vi "Measuring Complete - AndreTec-5-2.vi"() -> ()   [LabVIEW 2014]
doc: "André Romero - 2016\nandretec@ifsc.usp.br\nIFSC - USP"
uses:
  <vilib>/Analysis/Matrix/Datatypes/RealMatrix.ctl
  <vilib>/Analysis/Matrix/NI_Matrix.lvlib
  <vilib>/Instr/_visa.llb/VISA Configure Serial Port (Instr).vi
  <vilib>/Utility/file.llb/Write To Spreadsheet File (DBL).vi
  C:/UserLabs/Andre/Nova-Autolab/Labview/Autolab SDK 1.11/EcoChemie.Autolab.Sdk.dll
  EcoChemie.Autolab.Sdk.dll
panel:
  out "Procedure array":path[](array[path])=[path "C:/Users/user/Documents/My Procedures 1.11/Procedures/bla.nox", path "C:/Users/user/Documents/My Procedures 1.11/Procedures/bla2.nox", path "", path "", path "", path "", path "", path ""]
  in  "Tab Control":enum32{"Settings", "Measuring..."}(tab)
  in  "Load Procedure #8":path
  in  "Load Procedure #7":path
  in  "Load Procedure #6":path
  in  "Load Procedure #5":path
  in  "Load Procedure #4":path
  in  "Load Procedure #3":path
  in  "Load Procedure #2":path=path "C:/Users/user/Documents/My Procedures 1.11/Procedures/bla2.nox"
  in  "Load Procedure #1":path=path "C:/Users/user/Documents/My Procedures 1.11/Procedures/bla.nox"
  in  "Start Measurement":bool
  in  "X axis Sensor 1":string(combo)="WE(1).Potential"
  in  "Y axis Sersor 1":string(combo)="WE(1).Current"
  in  "X axis Sensor 2":string(combo)="WE(1).Potential"
  in  "Y axis Sersor 2":string(combo)="WE(1).Current"
  in  "X axis Sensor 3":string(combo)="WE(1).Potential"
  in  "Y axis Sersor 3":string(combo)="WE(1).Current"
  in  "X axis Sensor 4":string(combo)="WE(1).Potential"
  in  "Y axis Sersor 4":string(combo)="WE(1).Current"
  in  "X axis Sensor 5":string(combo)="WE(1).Potential"
  in  "Y axis Sersor 5":string(combo)="WE(1).Current"
  in  "X axis Sensor 6":string(combo)="WE(1).Potential"
  in  "Y axis Sersor 6":string(combo)="WE(1).Current"
  in  "X axis Sensor 7":string(combo)="WE(1).Potential"
  in  "Y axis Sersor 7":string(combo)="WE(1).Current"
  in  "X axis Sensor 8":string(combo)="WE(1).Potential"
  in  "Y axis Sersor 8":string(combo)="WE(1).Current"
  out "Measured data":cluster{"Y":dbl[], "Y":dbl[]}[](graph)=[{"Y"=[7.324218750000278e-05, 7.324218750000278e-05, 7.324218750000278e-05, 7.324218750000278e-05, 7.324218750000278e-05, 7.324218750000278e-05, 7.324218750000278e-05, 7.324218750000278e-05, 7.324218750000278e-05, 7.324218750000278e-05, 7.324218750000278e-05, 7.324218750000278e-05, 7.324218750000278e-05, 7.324218750000278e-05, 7.324218750000278e-05, 7.324218750000278e-05, 7.324218750000278e-05, 7.324218750000278e-05, 7.324218750000278e-05, 7.324218750000278e-05, 7.324218750000278e-05, 7.324218750000278e-05, 7.324218750000278e-05, 7.324218750000278e-05, 7.324218750000278e-05, 7.324218750000278e-05, 7.324218750000278e-05, 7.324218750000278e-05, 7.324218750000278e-05, 7.324218750000278e-05, 7.324218750000278e-05, 7.324218750000278e-05, 3.967285156250555e-05, 0.007351684570312503, 0.0195159912109375, 0.026904296874999997, 0.039157104492187504, 0.048931884765625, 0.06103515625, 0.068450927734375, 0.078125, 0.095245361328125, 0.10504150390625, 0.114776611328125, 0.1246337890625, 0.1343994140625, 0.144134521484375, 0.156402587890625, 0.163787841796875, 0.173431396484375, 0.185821533203125, 0.193084716796875, 0.205322265625, 0.215057373046875, 0.224945068359375, 0.234649658203125, 0.244384765625, 0.254180908203125, 0.266448974609375, 0.27386474609375, 0.285980224609375, 0.293365478515625, 0.30560302734375, 0.315277099609375, 0.32525634765625, 0.33502197265625, 0.347259521484375, 0.354461669921875, 0.364288330078125, 0.3765869140625, 0.38623046875, 0.396148681640625, 0.40594482421875, 0.415618896484375, 0.42791748046875, 0.435302734375, 0.447540283203125, 0.45477294921875, 0.467041015625, 0.474395751953125, 0.4864501953125, 0.4864501953125, 0.4864501953125, 0.4864501953125, 0.4864501953125, 0.4864501953125, 0.4864501953125, 0.4864501953125, 0.4864501953125, 0.4864501953125, 0.4864501953125, 0.4864501953125, 0.4864501953125, 0.4864501953125, 0.4864501953125, 0.4864501953125, 0.4864501953125, 0.4864501953125, 0.4864501953125, 0.4864501953125, 0.4864501953125, 0.4864501953125, 0.4864501953125, 0.4864501953125, 0.4864501953125, 0.4864501953125, 0.4864501953125, 0.4864501953125, 0.4864501953125, 0.4864501953125, 0.4864501953125, 0.4864501953125, 0.4864501953125, 0.4864501953125, 0.4864501953125, 0.4864501953125, 0.4864501953125, 0.4864501953125, 0.4864501953125, 0.4864501953125, 0.4864501953125, 0.4864501953125, 0.4864501953125, 0.4864501953125, 0.4864501953125, 0.4864501953125], "Y"=[-1.5228271484375027e-09, -1.5228271484375027e-09, -1.5228271484375027e-09, -1.5228271484375027e-09, -1.5228271484375027e-09, -1.5228271484375027e-09, -1.5228271484375027e-09, -1.5228271484375027e-09, -1.5228271484375027e-09, -1.5228271484375027e-09, -1.5228271484375027e-09, -1.5228271484375027e-09, -1.5228271484375027e-09, -1.5228271484375027e-09, -1.5228271484375027e-09, -1.5228271484375027e-09, -1.5228271484375027e-09, -1.5228271484375027e-09, -1.5228271484375027e-09, -1.5228271484375027e-09, -1.5228271484375027e-09, -1.5228271484375027e-09, -1.5228271484375027e-09, -1.5228271484375027e-09, -1.5228271484375027e-09, -1.5228271484375027e-09, -1.5228271484375027e-09, -1.5228271484375027e-09, -1.5228271484375027e-09, -1.5228271484375027e-09, -1.5228271484375027e-09, -1.5228271484375027e-09, 1.2298583984375e-09, 8.026123046875e-09, 2.056884765625e-08, 2.8045654296875e-08, 4.3182373046875e-08, 5.0750732421875e-08, 6.0791015625e-08, 7.302856445312499e-08, 8.0780029296875e-08, 9.7625732421875e-08, 1.02691650390625e-07, 1.1566162109375e-07, 1.23779296875e-07, 1.3873291015625e-07, 1.4031982421875e-07, 1.5744018554687499e-07, 1.6473388671875e-07, 1.7724609375e-07, 1.8524169921875e-07, 1.97265625e-07, 2.03948974609375e-07, 2.15118408203125e-07, 2.2833251953125e-07, 2.3315429687499998e-07, 2.47528076171875e-07, 2.5543212890624997e-07, 2.6641845703125e-07, 2.72979736328125e-07, 2.86376953125e-07, 2.97393798828125e-07, 3.0657958984375e-07, 3.16162109375e-07, 3.27911376953125e-07, 3.33251953125e-07, 3.4716796874999997e-07, 3.55987548828125e-07, 3.6611938476562497e-07, 3.74664306640625e-07, 3.900146484375e-07, 3.9682006835937497e-07, 4.1180419921874997e-07, 4.16595458984375e-07, 4.2974853515624997e-07, 4.3438720703125e-07, 4.505615234375e-07, 4.55657958984375e-07, 4.6716308593749996e-07, 4.7686767578125e-07, 4.91546630859375e-07, 4.91546630859375e-07, 4.91546630859375e-07, 4.91546630859375e-07, 4.91546630859375e-07, 4.91546630859375e-07, 4.91546630859375e-07, 4.91546630859375e-07, 4.91546630859375e-07, 4.91546630859375e-07, 4.91546630859375e-07, 4.91546630859375e-07, 4.91546630859375e-07, 4.91546630859375e-07, 4.91546630859375e-07, 4.91546630859375e-07, 4.91546630859375e-07, 4.91546630859375e-07, 4.91546630859375e-07, 4.91546630859375e-07, 4.91546630859375e-07, 4.91546630859375e-07, 4.91546630859375e-07, 4.91546630859375e-07, 4.91546630859375e-07, 4.91546630859375e-07, 4.91546630859375e-07, 4.91546630859375e-07, 4.91546630859375e-07, 4.91546630859375e-07, 4.91546630859375e-07, 4.91546630859375e-07, 4.91546630859375e-07, 4.91546630859375e-07, 4.91546630859375e-07, 4.91546630859375e-07, 4.91546630859375e-07, 4.91546630859375e-07, 4.91546630859375e-07, 4.91546630859375e-07, 4.91546630859375e-07, 4.91546630859375e-07, 4.91546630859375e-07, 4.91546630859375e-07, 4.91546630859375e-07, 4.91546630859375e-07]}]
  out "Autolab Connected":bool
  out "Blacklisted Commands detected":bool
  out "Y axis value":dbl=4.91546630859375e-07
  out "X axis value":dbl=0.4864501953125
  in  "X axis Signal":string(combo)="WE(1).Potential"
  in  "Y axis Signal":string(combo)="WE(1).Current"
  out "Points":i32=30
  out "Sensor":i32=2
  out "Measurement active":bool
  in  "Abort":bool
  in  "String":string="Wait !!!! Instrument is initializing ...."
  out "Measurement":cluster{dbl[], dbl[]}(graph)={[0.4864501953125, 0.4864501953125, 0.4864501953125, 0.4864501953125, 0.4864501953125, 0.4864501953125, 0.4864501953125, 0.4864501953125, 0.4864501953125, 0.4864501953125, 0.4864501953125, 0.4864501953125, 0.4864501953125, 0.4864501953125, 0.4864501953125, 0.4864501953125, 0.4864501953125, 0.4864501953125, 0.4864501953125, 0.4864501953125, 0.4864501953125, 0.4864501953125, 0.4864501953125, 0.4864501953125, 0.4864501953125, 0.4864501953125, 0.4864501953125, 0.4864501953125, 0.4864501953125, 0.4864501953125, 0.4864501953125], [4.91546630859375e-07, 4.91546630859375e-07, 4.91546630859375e-07, 4.91546630859375e-07, 4.91546630859375e-07, 4.91546630859375e-07, 4.91546630859375e-07, 4.91546630859375e-07, 4.91546630859375e-07, 4.91546630859375e-07, 4.91546630859375e-07, 4.91546630859375e-07, 4.91546630859375e-07, 4.91546630859375e-07, 4.91546630859375e-07, 4.91546630859375e-07, 4.91546630859375e-07, 4.91546630859375e-07, 4.91546630859375e-07, 4.91546630859375e-07, 4.91546630859375e-07, 4.91546630859375e-07, 4.91546630859375e-07, 4.91546630859375e-07, 4.91546630859375e-07, 4.91546630859375e-07, 4.91546630859375e-07, 4.91546630859375e-07, 4.91546630859375e-07, 4.91546630859375e-07, 4.91546630859375e-07]}
  out "error out":errorcluster
  out "VISA resource name out":refnum<visa-resource-name>="ASRL3::INSTR"
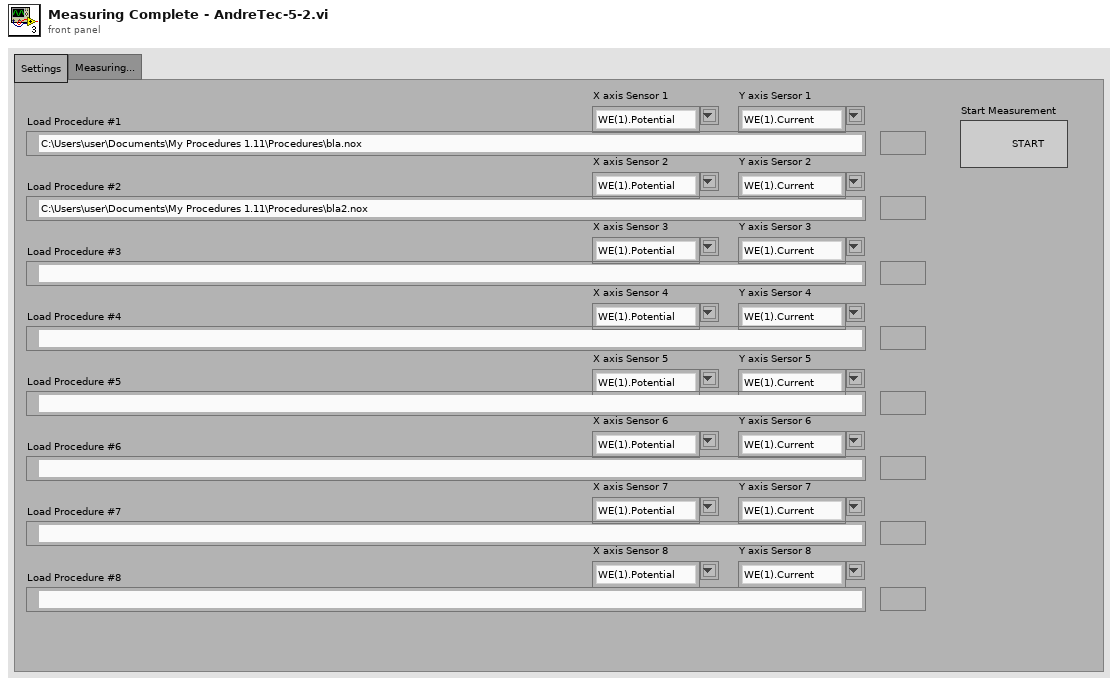
[diagram p1: front panel]
types:
  T1 = typedef "NI_Matrix.lvlib/RealMatrix.ctl" = dbl[][]
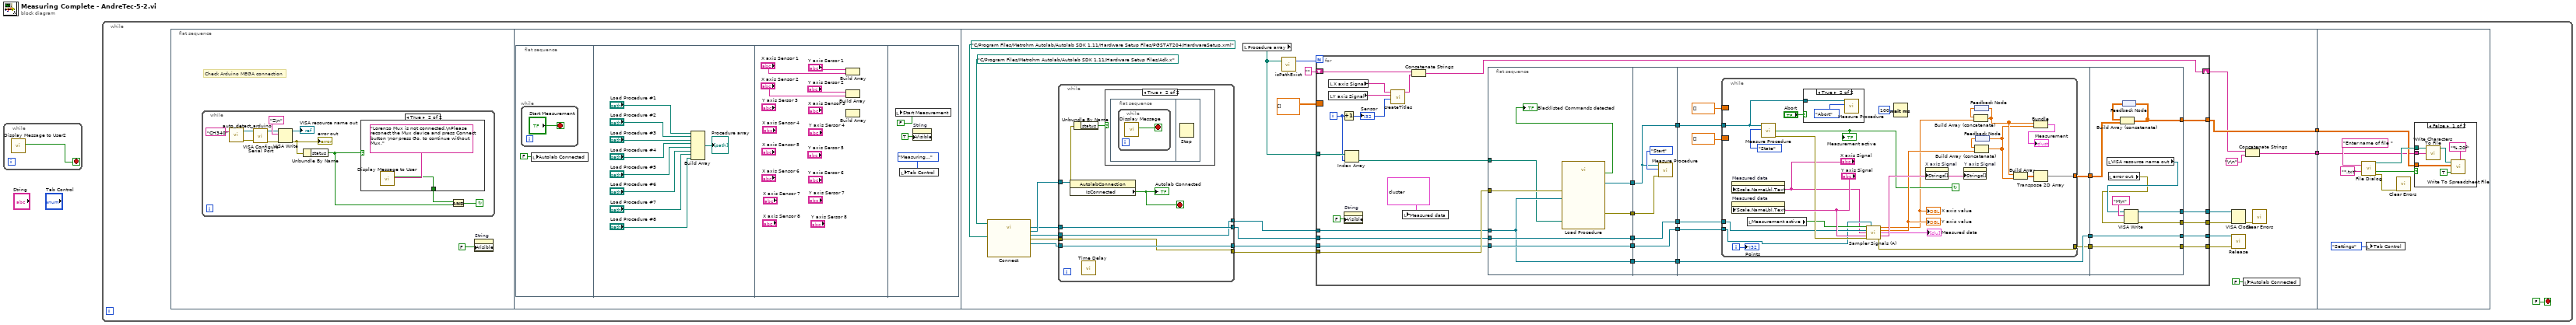
[diagram p0: block diagram]
diagram:
  n1 = while {
    stop <- w1 stop-if-true
    n2 = call "Display Message to User2"() -> ("OK"=w1:bool)  [unwired: 10 in, 1 out]
  }
  n3 = while {
    stop <- FALSE stop-if-true
    n4 = flat-sequence {
      tunnel: [w42] -> w3
      tunnel: [w40] -> w2
      tunnel: w3 -> [w163]
      tunnel: w2 -> [w162]
      frame #0 {
        # "Check Arduino MEGA connection"
        n5 = while {
          stop <- w8 continue-if-true
          n6 = call "auto_detect_arduino.vi"("instr name"="CH340") -> ("VISA resource name"=w16:refnum<visa-resource-name>, "error out"=w9:errorcluster)  [unwired: 1 in, 1 out]
          n7 = call-poly "VISA Configure Serial Port"("VISA resource name"=w16, "error in (no error)"=w9) -> ("VISA resource name out"=w13:refnum<visa-resource-name>, "error out"=w12:errorcluster)  [unwired: 7 in, 5 out]
          n8 = VISA Write(VISA resource name=w13, write buffer="Z\n" ("Command"), error in (no error)=w12) -> (VISA resource name out=→"VISA resource name out":refnum<visa-resource-name>, error out=w10:errorcluster)  [unwired: 1 out]
          "error out" <- w10
          n9 = Unbundle By Name(w10) -> ("status"=w7:bool)
          n10 = case shown="True" w7 {
            tunnel: [_ w17] -> w6
            frame False {
            }
            frame True {
              n11 = call "Display Message to User"("Message"="Lorenzo Mux is not connected.\nPlease reconect the Mux device and press Connect button \nor press Go, to continue without Mux.") -> ("Connect"=w17:bool)  [unwired: 9 in, 1 out]
            }
          }
          n12 = And(x=w6, y=w7) -> (x .and. y?=w8:bool)
        }
        n13 = property on="String" class="Str"("Visible"=FALSE) -> ()  [unwired: 2 in, 2 out]
      }
      frame #1 {
        n14 = flat-sequence {
          frame #0 {
            n15 = while {
              stop <- "Start Measurement" stop-if-true
            }
            n16 = local write "Autolab Connected"(FALSE ("Autolab Connected")) -> ()
          }
          frame #1 {
            n17 = Build Array("Load Procedure #1", "Load Procedure #2", "Load Procedure #3", "Load Procedure #4", "Load Procedure #5", "Load Procedure #6", "Load Procedure #7", "Load Procedure #8") -> (→"Procedure array":path[])
          }
          frame #2 {
            n18 = Build Array("Y axis Sersor 2", "X axis Sensor 2") -> ()  [unwired: 1 out]
            n19 = Build Array("Y axis Sersor 1", "X axis Sensor 1") -> ()  [unwired: 1 out]
            n20 = Build Array() -> ()  [unwired: 2 in, 1 out]
          }
          frame #3 {
            n21 = local write "Start Measurement"(FALSE ("Start Measurement")) -> ()
            n22 = local write "Tab Control"(enum32{"Settings", "Measuring..."}."Measuring..." ("Tab Control")) -> ()
            n23 = property on="String" class="Str"("Visible"=TRUE) -> ()  [unwired: 2 in, 2 out]
          }
        }
      }
      frame #2 {
        n24 = call "Connect.vi"("Embedded Exe File"=path "C:/Program Files/Metrohm Autolab/Autolab SDK 1.11/Hardware Setup Files/Adk.x", "Hardware Setup File"=path "C:/Program Files/Metrohm Autolab/Autolab SDK 1.11/Hardware Setup Files/PGSTAT204/HardwareSetup.xml") -> ("Sampler"=w58:refnum<k24>, "AutolabConnection"=w59:refnum<k24>, "instrument"=w56:refnum<k24>, "Ei"=w51:refnum<k24>, "error out"=w53:errorcluster)  [unwired: 1 in, 8 out]
        n25 = while {
          tunnel: w59 -> [w158]
          tunnel: w58 -> [w155]
          tunnel: [w155] -> w57
          tunnel: w56 -> [w154]
          tunnel: [w154] -> w55
          tunnel: w51 -> [w153]
          tunnel: [w153] -> w54
          tunnel: w53 -> [w152]
          tunnel: [w152] -> w52
          stop <- w159 stop-if-true
          n26 = property class="AutolabConnection"(reference=w158) -> (error out=w156:errorcluster, "IsConnected"=w159:bool)  [unwired: 1 in, 1 out]
          "Autolab Connected" <- w159
          n27 = Unbundle By Name(w156) -> ("status"=w157:bool)
          n28 = call "Time Delay"() -> ()  [unwired: 2 in, 10 out]
          n29 = case shown="True" w157 {
            frame False {
            }
            frame True {
              n30 = flat-sequence {
                frame #0 {
                  n31 = while {
                    stop <- w160 stop-if-true
                    n32 = call "Display Message"() -> ("OK"=w160:bool)  [unwired: 10 in, 1 out]
                  }
                }
                frame #1 {
                  n33 = Stop() -> ()  [unwired: 1 in]
                }
              }
            }
          }
        }
        n34 = local read "Procedure array"() -> (w37:path[])
        n35 = call "isPathExist.vi"("Array"=w37) -> ("Numeric"=w38:i16)  [unwired: 2 in]
        n36 = for {
          N: w38 -> [_]
          tunnel: [w82] -> w50
          tunnel: [w81] -> w49
          tunnel: [w80] -> w47
          tunnel: [w79] -> w46
          tunnel: w52 -> [w78]
          tunnel: w55 -> [w77]
          tunnel: w57 -> [w76]
          tunnel: w54 -> [w75]
          tunnel: [w73] -> w42
          border: T1 [] ("Real Matrix") -> [_]
          shift-right: [w70] -> w41
          shift-left: "" -> [w71]
          tunnel: w37 -> [w65]
          i -> [w64]
          n37 = local read "Y axis Signal"() -> (w68:string)
          n38 = local read "X axis Signal"() -> (w69:string)
          n39 = Increment(x=w64) -> (x+1=w67:i32)
          "Sensor" <- w67
          n40 = property on="String" class="Str"("Visible"=FALSE) -> ()  [unwired: 2 in, 2 out]
          n41 = Index Array(array=w65, index=w64) -> (element=w63:path)
          n42 = call "createTitles.vi"("Numeric"=w67, "Y axis Signal"=w68, "X axis Signal"=w69) -> ("String"=w66:string)  [unwired: 8 in]
          n43 = local write "Measured data"(cluster{"Y":dbl[], "Y":dbl[]}[] [{"Y"=array[2393 elements], "Y"=array[2393 elements]}] ("Measured data")) -> ()
          n44 = Concatenate Strings(w71, w66) -> (w70:string)
          n45 = flat-sequence {
            tunnel: [w100] -> w93
            tunnel: [w99] -> w92
            tunnel: [w97] -> w91
            tunnel: [w96] -> w90
            tunnel: [w95] -> w89
            tunnel: w77 -> [w95]
            tunnel: w78 -> [w98]
            tunnel: w76 -> [w97]
            tunnel: w75 -> [w96]
            tunnel: w63 -> [w94]
            tunnel: w93 -> [w105]
            tunnel: w92 -> [w106]
            tunnel: [w105] -> w88
            tunnel: w91 -> [w104]
            tunnel: w90 -> [w103]
            tunnel: [w104] -> w87
            tunnel: [w103] -> w86
            tunnel: [w102] -> w85
            tunnel: w89 -> [w102]
            tunnel: w88 -> [w115]
            tunnel: w87 -> [w114]
            tunnel: w86 -> [w113]
            tunnel: w85 -> [w112]
            tunnel: [w112] -> w84
            tunnel: [w108] -> w83
            tunnel: [w111] -> w74
            tunnel: w84 -> [w151]
            tunnel: w83 -> [w150]
            tunnel: [w151] -> w82
            tunnel: [w150] -> w81
            tunnel: [w146] -> w80
            tunnel: [w145] -> w79
            tunnel: w74 -> [w144]
            tunnel: [w142] -> w73
            frame #0 {
              n46 = call "Load Procedure.vi"("error in (no error)"=w98, "Procedure"=w94, "Instrument"=w95) -> ("error out"=w99:errorcluster, "Contains"=→"Blacklisted Commands detected":bool, "LoadProcedure"=w100:refnum<k24>)  [unwired: 6 out]
            }
            frame #1 {
              n47 = call "Measure Procedure.vi"("error in"=w106, "Request for procedure"=enum16{"State", "Save", "Abort", "Start"}."Start", "LoadProcedure"=w105) -> ()  [unwired: 1 in, 8 out]
            }
            frame #2 {
              n48 = while {
                tunnel: w115 -> [w132]
                tunnel: w114 -> [w133]
                tunnel: w113 -> [w117]
                tunnel: [w120] -> w111
                border: dbl[] [] -> [_]
                border: dbl[] [] -> [_]
                tunnel: [w119] -> w108
                i -> [w129]
                stop <- w124 continue-if-true
                n49 = property on="Measured data" class="XYGraph (strict)"("XScale.NameLbl.Text"="X axis Signal") -> ()  [unwired: 2 in, 2 out]
                n50 = property on="Measured data" class="XYGraph (strict)"("YScale.NameLbl.Text"="Y axis Signal") -> ()  [unwired: 2 in, 2 out]
                n51 = local read "Measurement active"() -> (w135:bool)
                n52 = call "Measure Procedure.vi"("Request for procedure"=enum16{"State", "Save", "Abort", "Start"}."State", "LoadProcedure"=w132) -> ("error out"=w136:errorcluster, "IsMeasuring"=w124:bool)  [unwired: 2 in, 6 out]
                "Measurement active" <- w124
                n53 = case shown="True" "Abort" {
                  tunnel: w132 -> [_ w140]
                  frame False {
                  }
                  frame True {
                    n54 = call "Measure Procedure.vi"("Request for procedure"=enum16{"State", "Save", "Abort", "Start"}."Abort", "LoadProcedure"=w140) -> ()  [unwired: 2 in, 8 out]
                  }
                }
                n55 = call "Sampler Signals (A).vi"("IsMeasuring"=w135, "EI"=w117, "Sampler"=w133, "Signal X"="X axis Signal", "Signal Y"="Y axis Signal", "error in"=w136) -> ("X"=w118:dbl, "Y"=w126:dbl, "XY Graph"=→"Measured data":cluster{"Y":dbl[], "Y":dbl[]}[], "GetSignals"=w138:string[], "error out"=w119:errorcluster)  [unwired: 4 in, 1 out]
                "Y axis value" <- w126
                "X axis value" <- w118
                n56 = Wait (ms)(milliseconds to wait=u32 100) -> ()  [unwired: 1 out]
                n57 = property on="X axis Signal" class="CmbBox"("Strings[]"=w138) -> ()  [unwired: 2 in, 2 out]
                n58 = property on="Y axis Signal" class="CmbBox"("Strings[]"=w138) -> ()  [unwired: 2 in, 2 out]
                n59 = feedback #1() -> (w128:dbl[])
                n60 = Build Array (concatenate)(w128, w118) -> (w122:dbl[])
                n61 = feedback-in #1(w122) -> ()
                n62 = feedback #2() -> (w127:dbl[])
                n63 = Build Array (concatenate)(w127, w126) -> (w121:dbl[])
                n64 = feedback-in #2(w121) -> ()
                n65 = Build Array(w122, w121) -> (w123:dbl[][])
                n66 = Bundle(w122, w121) -> (→"Measurement":cluster{dbl[], dbl[]})  [unwired: 1 in]
                n67 = Transpose 2D Array(2D array=w123) -> (transposed array=w120:dbl[][])
                "Points" <- w129
              }
            }
            frame #3 {
              n68 = local read "VISA resource name out"() -> (w148:refnum<visa-resource-name>)
              n69 = local read "error out"() -> (w147:errorcluster)
              n70 = feedback #3() -> (w143:T1)
              n71 = Build Array (concatenate)(w143, w144) -> (w142:T1)
              n72 = feedback-in #3(w142) -> ()
              n73 = VISA Write(VISA resource name=w148, write buffer="M\n" ("Command"), error in (no error)=w147) -> (VISA resource name out=w146:refnum<visa-resource-name>, error out=w145:errorcluster)  [unwired: 1 out]
            }
          }
        }
        n74 = call "Release.vi"("error in (no error)"=w49, "Instrument"=w50) -> ()  [unwired: 1 in, 9 out]
        n75 = VISA Close(VISA resource name=w47, error in (no error)=w46) -> (error out=w48:errorcluster)
        n76 = local write "Autolab Connected"(FALSE ("Autolab Connected")) -> ()
        n77 = Concatenate Strings(w41, "\r\n") -> (w40:string)
        n78 = call <vilib>:"Clear Errors.vi"("error in (no error)"=w48) -> ()  [unwired: 5 in, 2 out]
      }
      frame #3 {
        n79 = call "File Dialog"("prompt"="Enter name of file ", "pattern (all files)"="*.txt") -> ("selected path"=w166:path, "cancelled"=w164:bool, "error out"=w165:errorcluster)  [unwired: 10 in, 1 out]
        n80 = local write "Tab Control"(enum32{"Settings", "Measuring..."}."Settings" ("Tab Control")) -> ()
        n81 = call <vilib>:"Clear Errors.vi"("error in (no error)"=w165) -> ()  [unwired: 5 in, 2 out]
        n82 = case shown="False" w164 {
          tunnel: w166 -> [w174 _]
          tunnel: w163 -> [w171 _]
          tunnel: w162 -> [w170 _]
          frame False {
            n83 = call <vilib>:"Write Characters To File.vi"("character string"=w170, "file path (dialog if empty)"=w174) -> ("new file path (Not A Path if cancelled)"=w173:path)  [unwired: 3 in]
            n84 = call-poly <vilib>:"Write To Spreadsheet File.vi"("format (%.3f)"="%.20f", "append to file? (new file:F)"=TRUE, "2D data"=w171, "file path (dialog if empty)"=w173) -> ()  [unwired: 4 in, 1 out]
          }
          frame True {
          }
        }
      }
    }
  }
